vi "Create RxTx.vi"(8 "error in (no error)":errorcluster, 11 "Channel in":refnum<class "Channel.lvclass">) -> (0 "error out":errorcluster, 3 "Channel out":refnum<class "Channel.lvclass">)   [LabVIEW 2018, in "Channel.lvclass"]
uses:
  Channel.lvclass
  Channel.lvclass/Channel.ctl
  RxTx/RxTx.lvclass
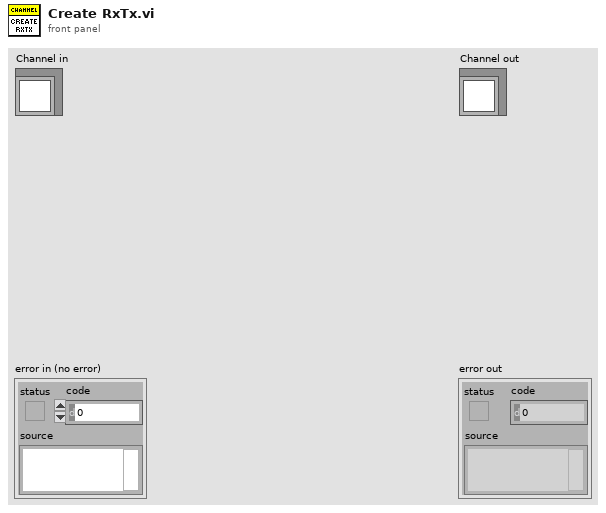
[diagram p1: front panel]
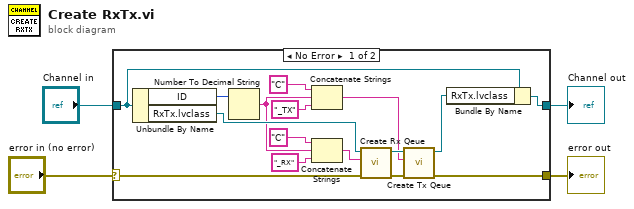
[diagram p0: block diagram]
diagram:
  n1 = case shown="No Error" "error in (no error)" {
    selector: "error in (no error)" -> [w18 w22]
    tunnel: [w20 w22] -> w3
    tunnel: [w14 w21] -> w1
    tunnel: "Channel in" -> [w15 w21]
    frame No Error {
      n2 = Unbundle By Name(w15) -> ("ID"=w5:u8, "RxTx.lvclass"=w17:refnum<class "RxTx.lvclass">)
      n3 = Number To Decimal String(number=w5) -> (decimal integer string=w7:string)  [unwired: 1 in]
      n4 = Concatenate Strings("C", w7, "_TX") -> (w6:string)
      n5 = Concatenate Strings("C", w7, "_RX") -> (w10:string)
      n6 = call "Create Rx Qeue.vi"("error in (no error)"=w18, "Reader Name"=w10, "RxTx in"=w17) -> ("error out"=w19:errorcluster, "RxTx out"=w16:refnum<class "RxTx.lvclass">)  [unwired: 7 in]
      n7 = call "Create Tx Qeue.vi"("error in (no error)"=w19, "Writer Name"=w6, "RxTx in"=w16) -> ("error out"=w20:errorcluster, "RxTx out"=w13:refnum<class "RxTx.lvclass">)  [unwired: 7 in]
      n8 = Bundle By Name(cluster=w15, "RxTx.lvclass"=w13) -> (w14:refnum<class "Channel.lvclass">)
    }
    frame Error {
    }
  }
  "error out" <- w3
  "Channel out" <- w1
